vi "Calculadora.vi"() -> ()   [LabVIEW 2020]
panel:
  in  "VALOR 1":enum16{""}(ring)
  in  "stop":bool
  out "Numeric 3":dbl
  in  "Enum":T1(ring) caption="OP BASICAS"
  in  "VALOR 2":dbl
  in  "VALOR 1":dbl
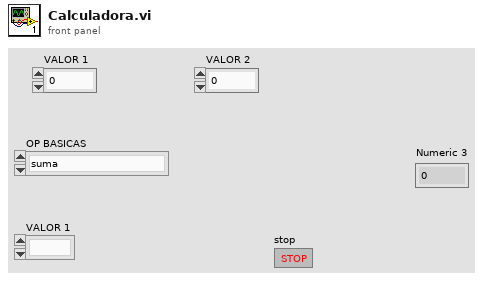
[diagram p1: front panel]
types:
  T1 = enum16{"suma", "resta", "multiplicacion", "division", "Pot. cuadrada VALOR 1", "Pot. Cuadrada VALOR 2", "Raiz Cuadrada VALOR 1", "Raiz Cuadrada VALOR 2"}
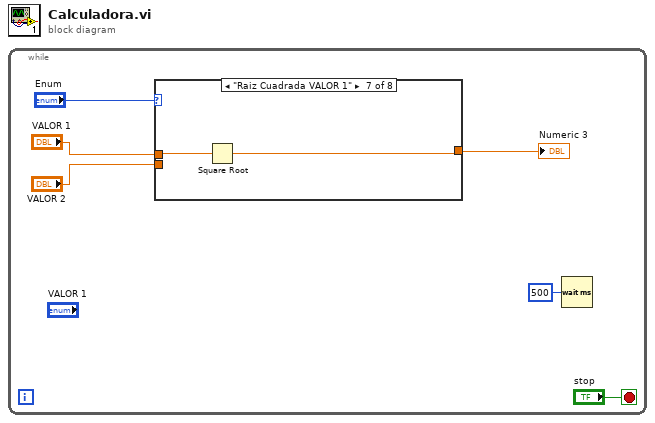
[diagram p0: block diagram]
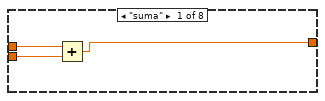
[diagram p2: hidden frame]
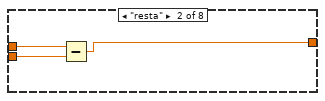
[diagram p3: hidden frame]
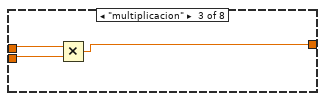
[diagram p4: hidden frame]
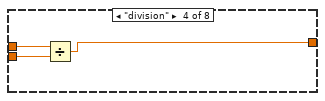
[diagram p5: hidden frame]
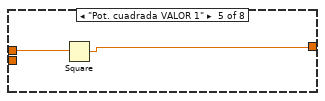
[diagram p6: hidden frame]
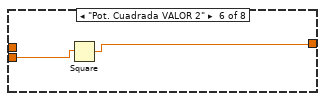
[diagram p7: hidden frame]
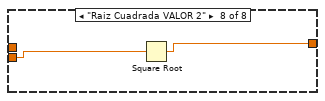
[diagram p8: hidden frame]
diagram:
  n1 = while {
    stop <- "stop" stop-if-true
    n2 = case shown="\"Raiz Cuadrada VALOR 1\"" "Enum" {
      tunnel: "VALOR 1" -> [w9 w12 w15 w18 w20 _ w24 _]
      tunnel: "VALOR 2" -> [w8 w11 w14 w17 _ w22 _ w26]
      tunnel: [w7 w10 w13 w16 w19 w21 w23 w25] -> w2
      frame "suma" {
        n3 = Add(x=w9, y=w8) -> (x+y=w7:dbl)
      }
      frame "resta" {
        n4 = Subtract(x=w12, y=w11) -> (x-y=w10:dbl)
      }
      frame "multiplicacion" {
        n5 = Multiply(x=w15, y=w14) -> (x*y=w13:dbl)
      }
      frame "division" {
        n6 = Divide(x=w18, y=w17) -> (x/y=w16:dbl)
      }
      frame "Pot. cuadrada VALOR 1" {
        n7 = Square(x=w20) -> (x^2=w19:dbl)
      }
      frame "Pot. Cuadrada VALOR 2" {
        n8 = Square(x=w22) -> (x^2=w21:dbl)
      }
      frame "Raiz Cuadrada VALOR 1" {
        n9 = Square Root(x=w24) -> (sqrt(x)=w23:dbl)
      }
      frame "Raiz Cuadrada VALOR 2" {
        n10 = Square Root(x=w26) -> (sqrt(x)=w25:dbl)
      }
    }
    "Numeric 3" <- w2
    n11 = Wait (ms)(milliseconds to wait=u32 500) -> ()  [unwired: 1 out]
  }
